vi "1.1 Drive Motor Limit.vi"(1 "Steer Direct":fxp<+/-,20,5>) -> (0 "Steering Limited":fxp<+/-,20,5>)   [LabVIEW 2010]
uses:
  1.0-Hindbrain Global.vi
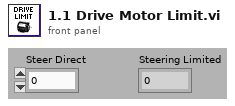
[diagram p1: front panel]
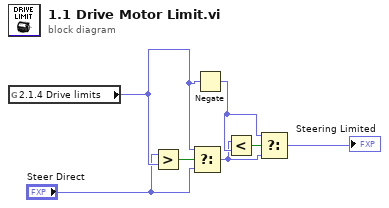
[diagram p0: block diagram]
diagram:
  n1 = global read "1.0-Hindbrain Global.vi" "2.1.4 Drive limits"() -> (w6:fxp<+/-,19,4>)
  n2 = Greater?(x="Steer Direct", y=w6) -> (0:w4:bool)
  n3 = Select(t=w6, s=w4, f="Steer Direct") -> (s? t:f=w1:fxp<+/-,20,5>)
  n4 = Negate(x=w6) -> (-x=w5:fxp<+/-,20,5>)
  n5 = Less?(x=w1, y=w5) -> (x < y?=w2:bool)
  n6 = Select(t=w5, s=w2, f=w1) -> (s? t:f=→"Steering Limited":fxp<+/-,20,5>)
